vi "EZ430-Chronos Error Generator.vi"(8 "Error In":errorcluster, 11 "EZ430-Chronos Error Code":i32) -> (0 "Error Out":errorcluster)   [LabVIEW 2011, in "LVH-EZ430.lvlib"]
uses:
  <vilib>/LabVIEW Hacker/LabVIEW Interface for EZ430-Chronos/LVH-EZ430.lvlib
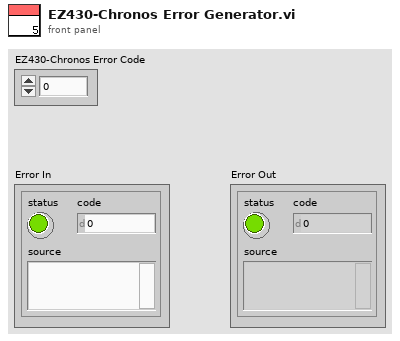
[diagram p1: front panel]
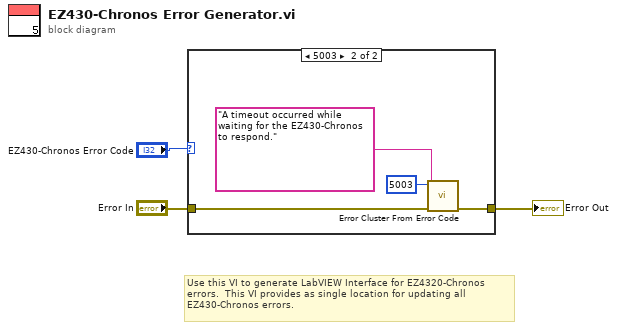
[diagram p0: block diagram]
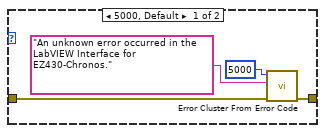
[diagram p2: hidden frame]
diagram:
  # "Use this VI to generate LabVIEW Interface for EZ4320-Chronos \nerrors.  This VI provides as single location for updating all \nEZ430-Chronos errors."
  n1 = case shown="5003" "EZ430-Chronos Error Code" {
    tunnel: "Error In" -> [w5 w9]
    tunnel: [w4 w10] -> w1
    frame 5000, Default {
      n2 = call <vilib>:"Error Cluster From Error Code.vi"("error in (no error)"=w5, "error message (\"\")"="An unknown error occurred in the LabVIEW Interface for EZ430-Chronos.", "error code (0)"=5000) -> ("error out"=w4:errorcluster)  [unwired: 6 in]
    }
    frame 5003 {
      n3 = call <vilib>:"Error Cluster From Error Code.vi"("error in (no error)"=w9, "error message (\"\")"="A timeout occurred while waiting for the EZ430-Chronos to respond." ("error message (\"\")"), "error code (0)"=5003) -> ("error out"=w10:errorcluster)  [unwired: 6 in]
    }
  }
  "Error Out" <- w1
